vi "Remove Connections from State.vi"(8 "error in (no error)":errorcluster, 10 "Connection List":T1[](array[typedef]), 11 "Routing State in":T2) -> (0 "error out":errorcluster, 1 "connection not found":bool, 3 "Routing State out":T2)   [LabVIEW 2017, in "Switch Scripting.lvlib"]
uses:
  Switch Scripting.lvlib
  Routing State.ctl
  Connection.ctl
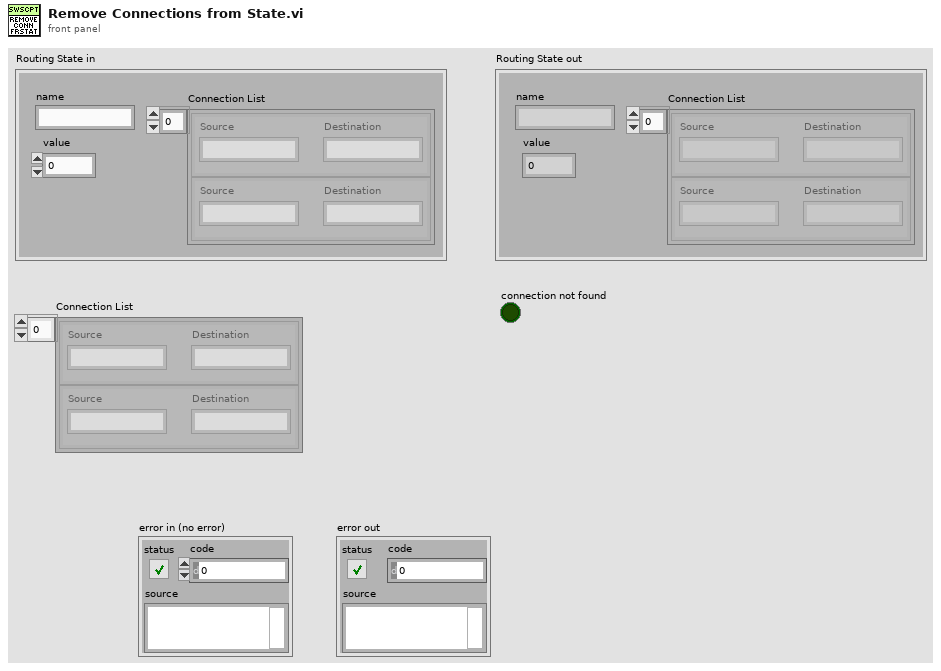
[diagram p1: front panel]
types:
  T1 = typedef "Switch Scripting.lvlib/Connection.ctl" = cluster{"Source":string, "Destination":string}
  T2 = typedef "Switch Scripting.lvlib/Routing State.ctl" = cluster{"name":string, "value":i32, "Connection List":T1[]}
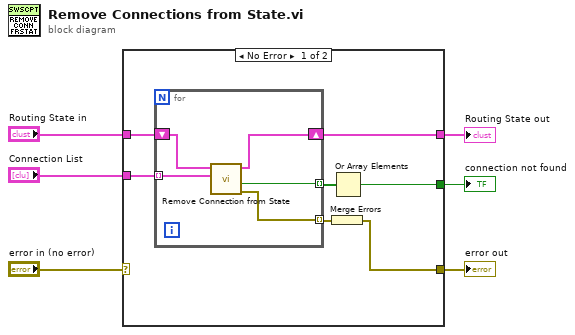
[diagram p0: block diagram]
diagram:
  n1 = case shown="No Error" "error in (no error)" {
    selector: "error in (no error)" -> [_ w20]
    tunnel: [w7 w20] -> w6
    tunnel: [w9 w19] -> w5
    tunnel: "Routing State in" -> [w11 w19]
    tunnel: "Connection List" -> [w10 _]
    tunnel: [w12 _] -> w1
    frame No Error {
      n2 = for {
        tunnel: [w18] -> w13 mode=indexing
        shift-right: [w16] -> w9
        shift-left: w11 -> [w17]
        tunnel: w10 -> [w15] mode=indexing
        tunnel: [w14] -> w8 mode=indexing
        n3 = call "Remove Connection from State.vi"("Connection"=w15, "Routing State in"=w17) -> ("error out"=w14:errorcluster, "connection not found"=w18:bool, "Routing State out"=w16:T2)  [unwired: 7 in]
      }
      n4 = Merge Errors(w8) -> (w7:errorcluster)
      n5 = Or Array Elements(Boolean array=w13) -> (logical OR=w12:bool)
    }
    frame Error {
    }
  }
  "error out" <- w6
  "Routing State out" <- w5
  "connection not found" <- w1
